vi "Write Heater.vi"(8 "error in (no error)":errorcluster, 10 "Heater":T1 max=100.0 scale=0.0..100.0 scale format="%.1f", 11 "Temperature Controller in":refnum<class "Temperature Controller.lvclass">) -> (0 "error out":errorcluster, 3 "Temperature Controller out":refnum<class "Temperature Controller.lvclass">)   [LabVIEW 2009, in "Temperature Controller.lvclass"]
uses:
  Temperature Controller.lvclass
  HV Slide Indicator.ctl
  Temperature Controller.lvclass/Temperature Controller.ctl
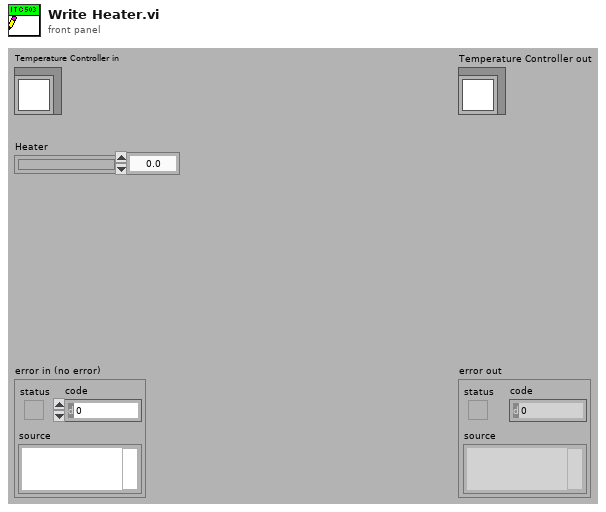
[diagram p1: front panel]
types:
  T1 = typedef "Temperature Controller.lvclass/HV Slide Indicator.ctl" = dbl
  T2 = typedef "ITCIO.ctl" = cluster{"Address":T3, "Version":T4, "Ch 1 dec places":i16, "Ch 2 dec places":i16, "Ch 3 dec places":i16, "Ch1 Name":string, "Ch2 Name":string, "Ch3 Name":string}
  T3 = typedef "OxfordAddress.ctl" = cluster{"Com Port":i32, "ISOBUS Address":i32, "GPIB Address":i16, "Communication":enum16{"RS232", "ISOBUS", "GPIB", "Gateway"}}
  T4 = typedef "ITCVersion.ctl" = enum16{"ITC502", "ITC503", "ITC601"}
  T5 = typedef "Temperature Controller.lvclass/AutoCtl.ctl" = cluster{"Auto Heater":bool, "Auto Needle":bool, "Auto PID":bool}
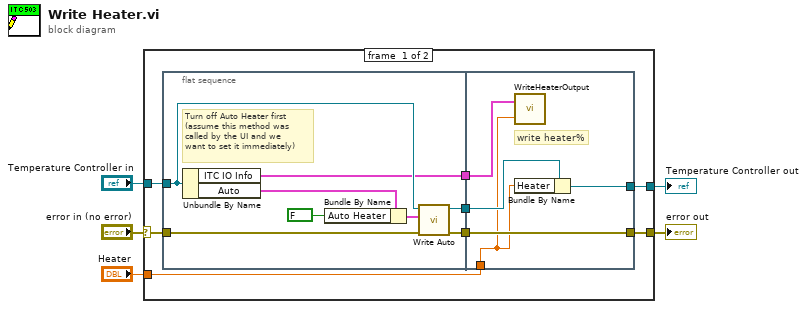
[diagram p0: block diagram]
diagram:
  n1 = case shown="No Error" "error in (no error)" {
    selector: "error in (no error)" -> [w12 w27]
    tunnel: [w11 w27] -> w4
    tunnel: [w6 w28] -> w2
    tunnel: "Temperature Controller in" -> [w13 w28]
    tunnel: "Heater" -> [w8 _]
    frame #0 {
      n2 = flat-sequence {
        tunnel: w13 -> [w18]
        tunnel: w12 -> [w21]
        tunnel: [w20] -> w10
        tunnel: [w17] -> w9
        tunnel: [w14] -> w7
        tunnel: [w26] -> w11
        tunnel: w10 -> [w26]
        tunnel: w8 -> [w22]
        tunnel: w9 -> [w25]
        tunnel: w7 -> [w24]
        tunnel: [w23] -> w6
        frame #0 {
          # "Turn off Auto Heater first\n(assume this method was\ncalled by the UI and we\nwant to set it immediately)"
          n3 = Unbundle By Name(w18) -> ("ITC IO Info"=w17:T2, "Auto"=w16:T5)
          n4 = Bundle By Name(cluster=w16, "Auto Heater"=FALSE ("Auto Needle")) -> (w15:T5)
          n5 = call-dynamic "Write Auto.vi"("error in (no error)"=w21, "Auto"=w15, "Temperature Controller in"=w18) -> ("error out"=w20:errorcluster, "Temperature Controller out"=w14:refnum<class "Temperature Controller.lvclass">)  [unwired: 7 in]
        }
        frame #1 {
          # "write heater%"
          n6 = call "WriteHeaterOutput.vi"("Heater Output (%)"=w22, "ITC IO Info"=w25) -> ()  [unwired: 2 out]
          n7 = Bundle By Name(cluster=w24, "Heater"=w22) -> (w23:refnum<class "Temperature Controller.lvclass">)
        }
      }
    }
    frame #1 {
    }
  }
  "error out" <- w4
  "Temperature Controller out" <- w2
